vi "TestQtyCheck.vi"() -> ()   [LabVIEW 2012]
uses:
  <vilib>/addons/database/Auxilliary.llb/DB Tools Cursor Type.ctl
  <vilib>/Utility/NIReport.llb/NI_report.lvclass
  <vilib>/addons/database/Connection.llb/DB Tools Open Connec (Path).vi
  <vilib>/addons/database/Connection.llb/Conn Execute.vi
  <vilib>/addons/database/Recordset.llb/Rec Fetch Recordset Data (R).vi
  <vilib>/addons/database/Recordset.llb/Rec Destroy - Connection.vi
  <vilib>/addons/database/Recordset.llb/Rec Fetch Integer Data (R).vi
  <vilib>/addons/database/Recordset.llb/Rec Fetch String Data (R).vi
  <vilib>/Utility/NIReport.llb/Append Text Table to Report (wrap).vi
  <vilib>/addons/database/_DB Variant To Data/Database Variant To Data.xnode
  <vilib>/addons/database/NI_Database_API.lvlib
  <vilib>/Utility/NIReport.llb/Excel/NI_Excel.lvclass
panel:
  out "concatenated string 2":string
  out "error out 3":errorcluster
  out "error out 2":errorcluster
  in  "template (empty)":path=path "O:/Monitor/Report/機台報表示數量確認LIST.xls"
  out "array":string[][](array[string])
  out "spreadsheet string":string
  out "String":string
  out "concatenated string":string
  out "data":string
  out "data 4":i32
  out "data 3":string
  out "data 2":i32
  out "error out":errorcluster
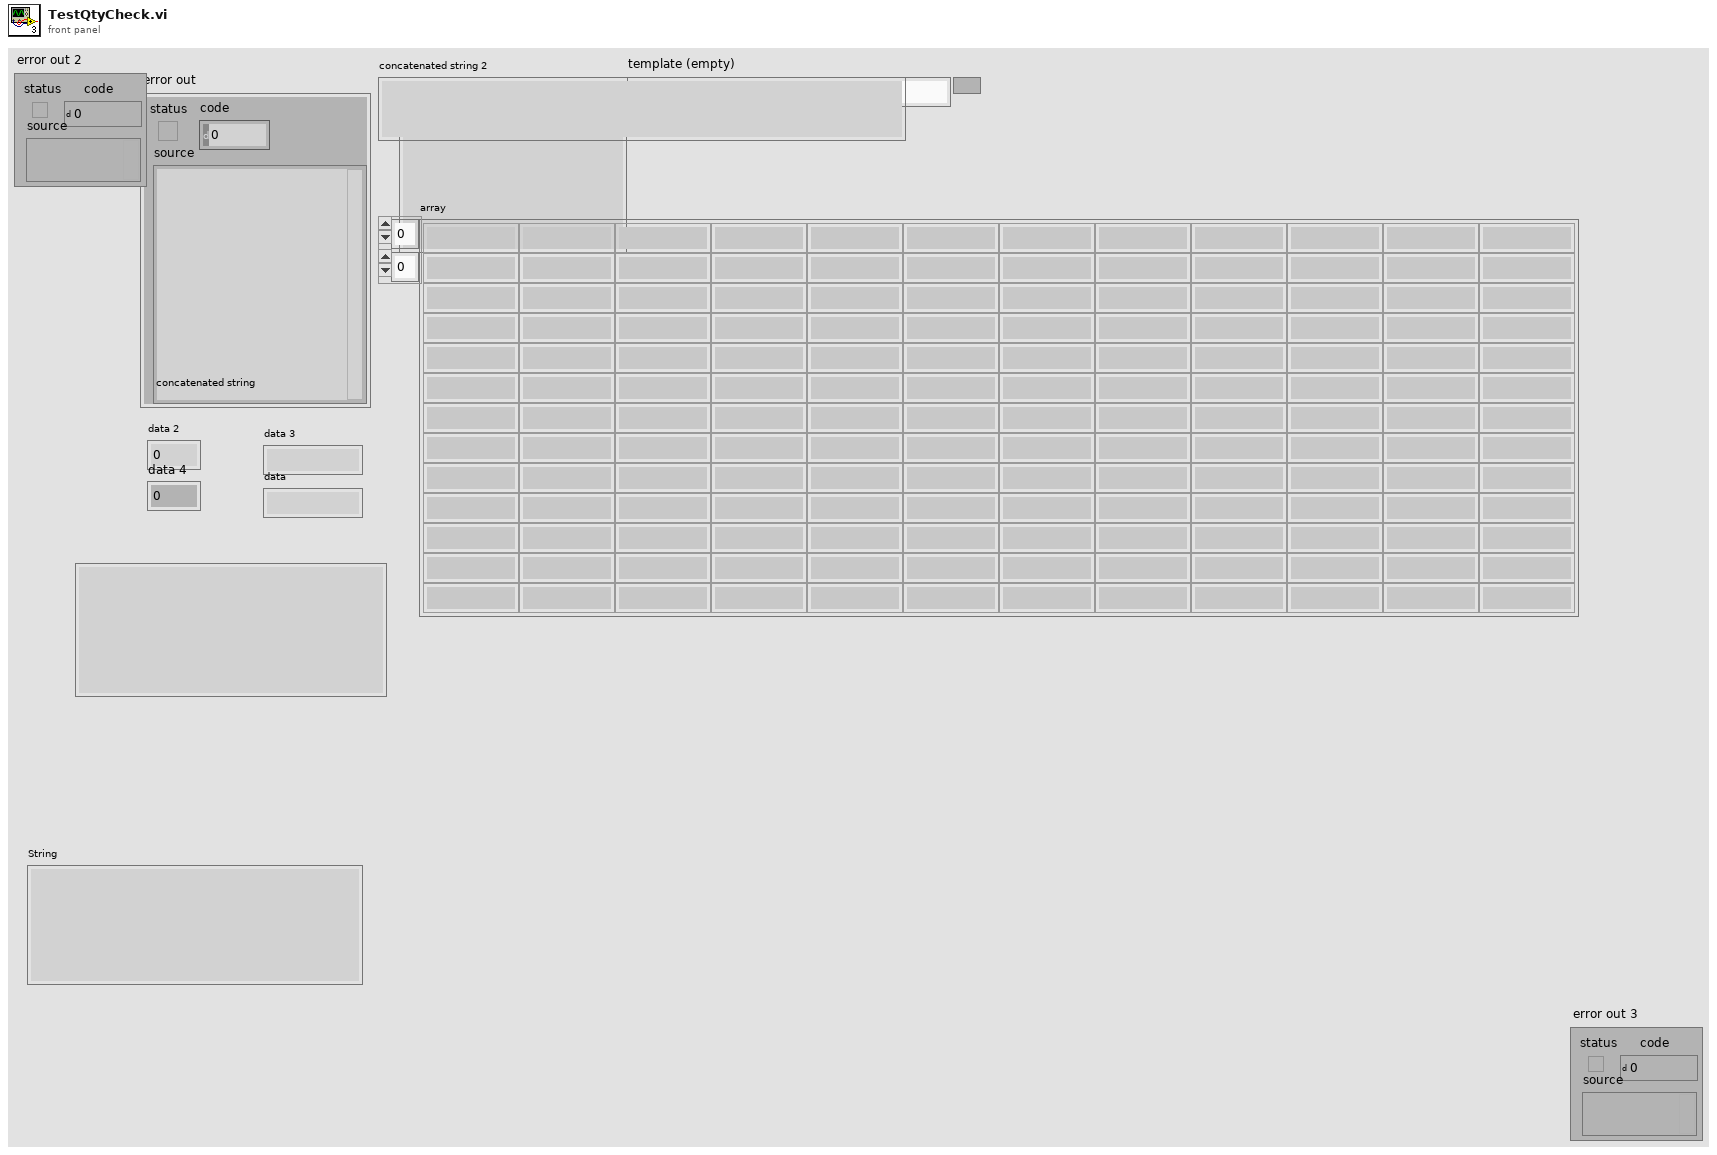
[diagram p1: front panel]
types:
  T1 = typedef "NI_Database_API.lvlib/DB Tools Cursor Type.ctl" = enum16{"forward-only", "keyset", "dynamic", "static"}
  T2 = typedef "NI_Database_API.lvlib/Conn ObjectReference.ctl" = refnum<k1>
  T3 = typedef "NI_Database_API.lvlib/Rec ObjectReference.ctl" = refnum<k1>
  T4 = enum16{"Standard Report", "HTML", "Word", "Excel"}
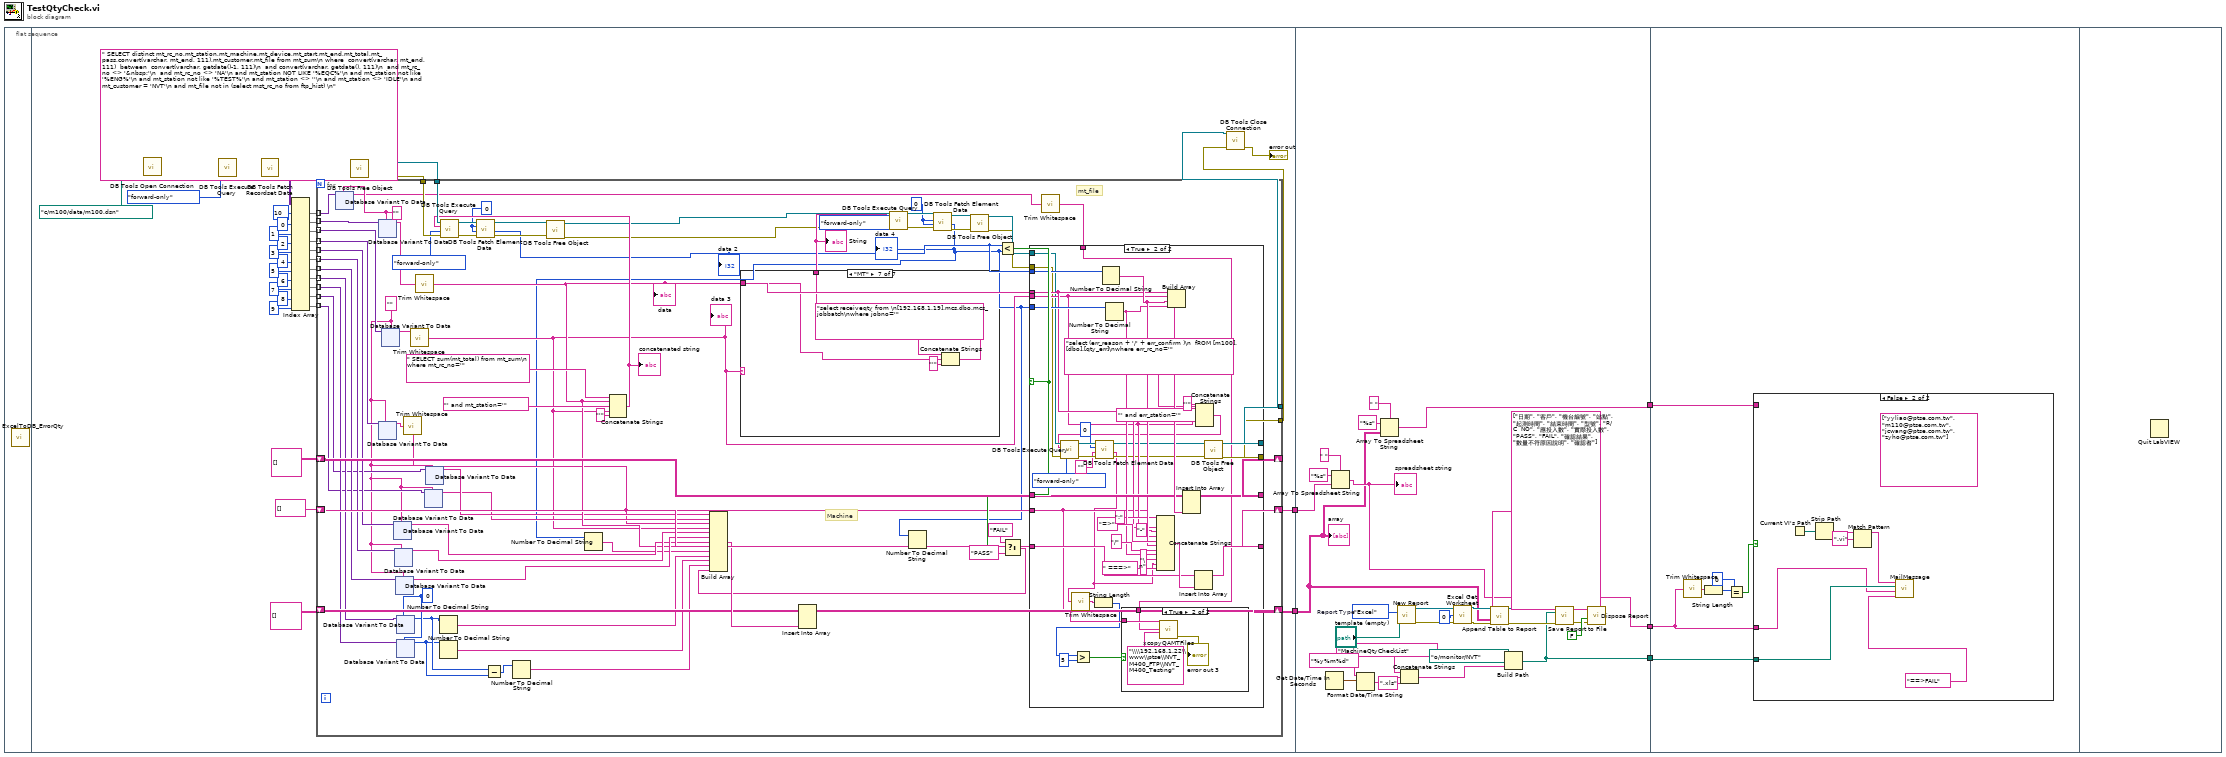
[diagram p0: block diagram]
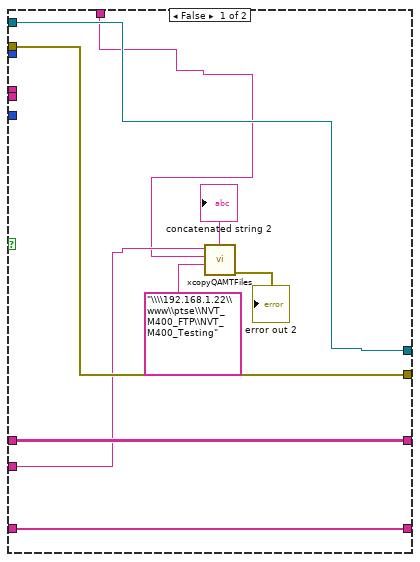
[diagram p2: hidden frame]
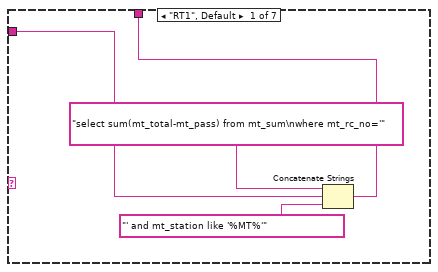
[diagram p4: hidden frame]
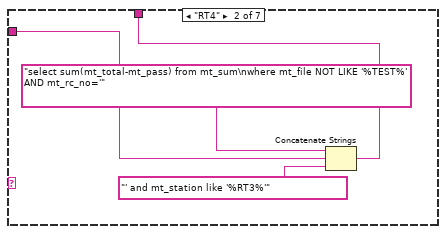
[diagram p5: hidden frame]
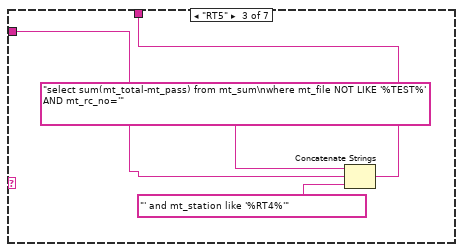
[diagram p6: hidden frame]
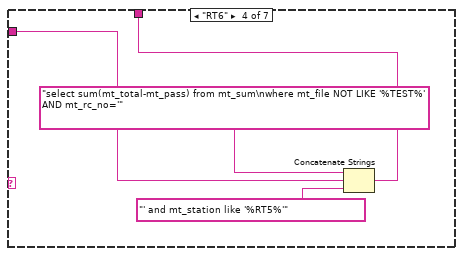
[diagram p7: hidden frame]
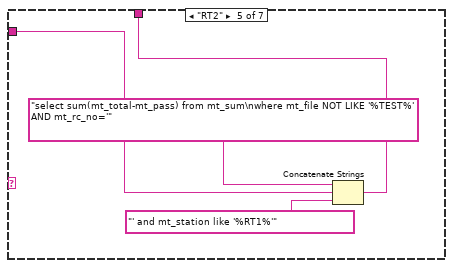
[diagram p8: hidden frame]
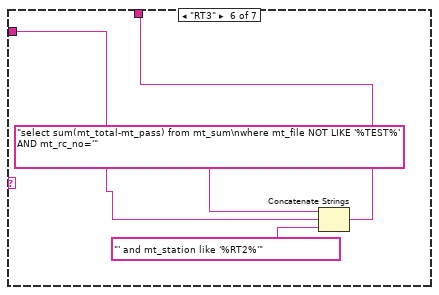
[diagram p9: hidden frame]
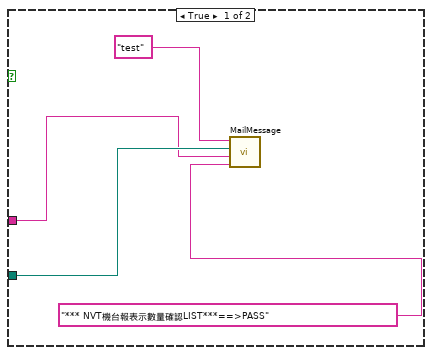
[diagram p10: hidden frame]
diagram:
  n1 = flat-sequence {
    tunnel: [w28] -> w5
    tunnel: [w24] -> w4
    tunnel: w5 -> [w579]
    tunnel: w4 -> [w555]
    tunnel: [w558] -> w3
    tunnel: [w557] -> w2
    tunnel: [w553] -> w1
    tunnel: w3 -> [w588]
    tunnel: w2 -> [w587]
    tunnel: w1 -> [w582]
    frame #0 {
      n2 = call "ExcelToDB_ErrorQty.vi"() -> ()  [unwired: 12 in]
    }
    frame #1 {
      n3 = call-poly <vilib>:"DB Tools Open Connection.vi"("connection information"=path "c:/m100/data/m100.dsn") -> ("error out"=w45:errorcluster, "connection reference"=w46:T2)  [unwired: 7 in]
      n4 = call-poly <vilib>:"DB Tools Execute Query.vi"("error in (no error)"=w45, "cursor type"=DB_Tools_Cursor_Type."forward-only", "SQL query"=" SELECT distinct mt_rc_no,mt_station,mt_machine,mt_device,mt_start,mt_end,mt_total,mt_pass,convert(varchar, mt_end, 111),mt_customer,mt_file from mt_sum\n where  convert(varchar, mt_end, 111)  between  convert(varchar, getdate()-1, 111)\n  and convert(varchar, getdate(), 111)\n  and mt_rc_no <> '&nbsp;'\n  and mt_rc_no <> 'NA'\n and mt_station NOT LIKE '%EQC%'\n and mt_station not like '%ENG%'\n and mt_station not like '%TEST%'\n and mt_station <> ''\n and mt_station <> 'IDLE'\n and mt_customer = 'NVT'\n and mt_file not in (select mst_rc_no from ftp_hist) \n", "connection reference"=w46) -> ("error out"=w43:errorcluster, "recordset reference"=w44:T3)  [unwired: 4 in]
      n5 = call-poly <vilib>:"DB Tools Fetch Recordset Data.vi"("error in (no error)"=w43, "recordset reference"=w44) -> ("error out"=w41:errorcluster, "recordset data"=w37:variant[][], "recordset reference out"=w42:T3)  [unwired: 3 in]
      n6 = Index Array(array=w37, index (col) #1=10 ("disabled index (col)"), index (col) #2=0 ("disabled index (col)"), index (col) #3=1 ("index (col)"), index (col) #4=2 ("index (col)"), index (col) #5=3 ("index (col)"), index (col) #6=4 ("index (col)"), index (col) #7=5 ("index (col)"), index (col) #8=6 ("index (col)"), index (col) #9=7 ("index (col)"), index (col) #10=8 ("index (col)"), index (col) #11=9 ("index (col)")) -> (element #1=w6:variant[], element #2=w36:variant[], element #3=w33:variant[], element #4=w26:variant[], element #5=w20:variant[], element #6=w19:variant[], element #7=w18:variant[], element #8=w15:variant[], element #9=w14:variant[], element #10=w11:variant[], element #11=w10:variant[])  [unwired: 11 in]
      n7 = call-poly <vilib>:"DB Tools Free Object.vi"("error in (no error)"=w41, "recordset reference"=w42) -> ("error out"=w31:errorcluster, "connection reference"=w32:T2)  [unwired: 8 in]
      n8 = for {
        tunnel: w36 -> [w111] mode=indexing
        tunnel: w33 -> [w119] mode=indexing
        tunnel: w32 -> [w110]
        tunnel: w31 -> [w109]
        shift-right: [w94] -> _
        shift-left: string[][] [] ("array") -> [w93]
        shift-right: [w54] -> w28
        shift-left: string[] [] ("array") -> [w92]
        tunnel: w26 -> [w91] mode=indexing
        shift-right: [w85] -> w24
        shift-left: string[][] [] ("array") -> [w83]
        tunnel: w20 -> [w82] mode=indexing
        tunnel: w19 -> [w81] mode=indexing
        tunnel: w18 -> [w80] mode=indexing
        tunnel: w15 -> [w79] mode=indexing
        tunnel: w14 -> [w78] mode=indexing
        tunnel: w11 -> [w73] mode=indexing
        tunnel: w10 -> [w72] mode=indexing
        tunnel: [w60] -> w9
        tunnel: [w59] -> w8
        tunnel: w6 -> [w58] mode=indexing
        w77 = 0
        w112 = 0
        w101 = 0
        w71 = ""
        w57 = ""
        # "Machine"
        # "mt_file"
        n9 = xnode "Database Variant To Data"("database variant"=w58, "type"=w57) -> ("data"=w56:string)  [unwired: 1 in, 1 out]
        n10 = xnode "Database Variant To Data"("database variant"=w91, "type"=w71) -> ("data"=w90:string)  [unwired: 1 in, 1 out]
        n11 = xnode "Database Variant To Data"("database variant"=w111, "type"=w57) -> ("data"=w95:string)  [unwired: 1 in, 1 out]
        n12 = xnode "Database Variant To Data"("database variant"=w119, "type"=w71) -> ("data"=w96:string)  [unwired: 1 in, 1 out]
        n13 = xnode "Database Variant To Data"("database variant"=w82, "type"=w71) -> ("data"=w68:string)  [unwired: 1 in, 1 out]
        n14 = xnode "Database Variant To Data"("database variant"=w81, "type"=w71) -> ("data"=w70:string)  [unwired: 1 in, 1 out]
        n15 = xnode "Database Variant To Data"("database variant"=w80, "type"=w71) -> ("data"=w69:string)  [unwired: 1 in, 1 out]
        n16 = xnode "Database Variant To Data"("database variant"=w79, "type"=w77) -> ("data"=w76:i32)  [unwired: 1 in, 1 out]
        n17 = xnode "Database Variant To Data"("database variant"=w78, "type"=w77) -> ("data"=w75:i32)  [unwired: 1 in, 1 out]
        n18 = call <vilib>:"Trim Whitespace.vi"("string"=w90) -> ("trimmed string"=w64:string)  [unwired: 1 in]
        n19 = call <vilib>:"Trim Whitespace.vi"("string"=w96) -> ("trimmed string"=w63:string)  [unwired: 1 in]
        "data 3" <- w63
        n20 = call <vilib>:"Trim Whitespace.vi"("string"=w95) -> ("trimmed string"=w67:string)  [unwired: 1 in]
        "data" <- w67
        n21 = xnode "Database Variant To Data"("database variant"=w72, "type"=w71) -> ("data"=w65:string)  [unwired: 1 in, 1 out]
        n22 = xnode "Database Variant To Data"("database variant"=w73, "type"=w71) -> ("data"=w66:string)  [unwired: 1 in, 1 out]
        n23 = Number To Decimal String(number=w76) -> (decimal integer string=w50:string)  [unwired: 1 in]
        n24 = Number To Decimal String(number=w75) -> (decimal integer string=w51:string)  [unwired: 1 in]
        n25 = Subtract(x=w76, y=w75) -> (x-y=w74:i32)
        n26 = Number To Decimal String(number=w74) -> (decimal integer string=w52:string)  [unwired: 1 in]
        n27 = Concatenate Strings(" SELECT sum(mt_total) from mt_sum\n where mt_rc_no='", w67, "' and mt_station='" ("string"), w63, "'" ("string")) -> (w102:string)
        "concatenated string" <- w102
        n28 = call-poly <vilib>:"DB Tools Execute Query.vi"("error in (no error)"=w109, "cursor type"=DB_Tools_Cursor_Type."forward-only", "SQL query"=w102, "connection reference"=w110) -> ("error out"=w107:errorcluster, "recordset reference"=w108:T3)  [unwired: 4 in]
        n29 = call-poly <vilib>:"DB Tools Fetch Element Data.vi"("error in (no error)"=w107, "type"=w101, "column index"=w101, "recordset reference"=w108) -> ("error out"=w99:errorcluster, "data"=w89:i32, "recordset reference out"=w100:T3)  [unwired: 3 in]
        "data 2" <- w89
        n30 = call-poly <vilib>:"DB Tools Free Object.vi"("error in (no error)"=w99, "recordset reference"=w100) -> ("error out"=w98:errorcluster, "connection reference"=w97:T2)  [unwired: 8 in]
        n31 = case shown="\"MT\"" w63 {
          tunnel: w67 -> [w462 w465 w469 w473 w478 w481 w487]
          tunnel: [w461 w466 w470 w474 w477 w482 w486] -> w114
          frame "RT1", Default {
            n32 = Concatenate Strings("select sum(mt_total-mt_pass) from mt_sum\nwhere mt_rc_no='" ("string"), w462, "' and mt_station like '%MT%'" ("string")) -> (w461:string)
          }
          frame "RT4" {
            n33 = Concatenate Strings("select sum(mt_total-mt_pass) from mt_sum\nwhere mt_file NOT LIKE '%TEST%' AND mt_rc_no='" ("string"), w465, "' and mt_station like '%RT3%'" ("string")) -> (w466:string)
          }
          frame "RT5" {
            n34 = Concatenate Strings("select sum(mt_total-mt_pass) from mt_sum\nwhere mt_file NOT LIKE '%TEST%' AND mt_rc_no='" ("string"), w469, "' and mt_station like '%RT4%'" ("string")) -> (w470:string)
          }
          frame "RT6" {
            n35 = Concatenate Strings("select sum(mt_total-mt_pass) from mt_sum\nwhere mt_file NOT LIKE '%TEST%' AND mt_rc_no='" ("string"), w473, "' and mt_station like '%RT5%'" ("string")) -> (w474:string)
          }
          frame "RT2" {
            n36 = Concatenate Strings("select sum(mt_total-mt_pass) from mt_sum\nwhere mt_file NOT LIKE '%TEST%' AND mt_rc_no='" ("string"), w478, "' and mt_station like '%RT1%'" ("string")) -> (w477:string)
          }
          frame "RT3" {
            n37 = Concatenate Strings("select sum(mt_total-mt_pass) from mt_sum\nwhere mt_file NOT LIKE '%TEST%' AND mt_rc_no='" ("string"), w481, "' and mt_station like '%RT2%'" ("string")) -> (w482:string)
          }
          frame "MT" {
            n38 = Concatenate Strings("select receiveqty from \n[192.168.1.19].mcs.dbo.mcs_jobbatch\nwhere jobno='" ("string"), w487, "'" ("string")) -> (w486:string)
          }
        }
        "String" <- w114
        n39 = call-poly <vilib>:"DB Tools Execute Query.vi"("error in (no error)"=w98, "cursor type"=DB_Tools_Cursor_Type."forward-only", "SQL query"=w114, "connection reference"=w97) -> ("error out"=w113:errorcluster, "recordset reference"=w117:T3)  [unwired: 4 in]
        n40 = call-poly <vilib>:"DB Tools Fetch Element Data.vi"("error in (no error)"=w113, "type"=w112, "column index"=w112, "recordset reference"=w117) -> ("error out"=w115:errorcluster, "data"=w49:i32, "recordset reference out"=w116:T3)  [unwired: 3 in]
        "data 4" <- w49
        n41 = Number To Decimal String(number=w49) -> (decimal integer string=w48:string)  [unwired: 1 in]
        n42 = Number To Decimal String(number=w49) -> ()  [unwired: 1 in, 1 out]
        n43 = call-poly <vilib>:"DB Tools Free Object.vi"("error in (no error)"=w115, "recordset reference"=w116) -> ("error out"=w61:errorcluster, "connection reference"=w62:T2)  [unwired: 8 in]
        n44 = Less?(x=w89, y=w49) -> (x < y?=w88:bool)
        n45 = Select(t="FAIL", s=w88, f="PASS") -> (s? t:f=w53:string)
        n46 = Build Array(w66, w65, w64, w63, w70, w69, w68, w67, w48, w50, w51, w52, w53) -> (w84:string[])
        n47 = Insert Into Array(array=w83, new element=w84) -> (w85:string[][])  [unwired: 2 in]
        n48 = call <vilib>:"Trim Whitespace.vi"("string"=w56) -> ("trimmed string"=w55:string)  [unwired: 1 in]
        n49 = case shown="True" w88 {
          tunnel: w67 -> [_ w441]
          tunnel: w63 -> [_ w439]
          tunnel: w89 -> [_ w456]
          tunnel: w49 -> [_ w455]
          tunnel: [w416 w453] -> w94
          tunnel: w93 -> [w416 w452]
          tunnel: [w415 w446] -> w54
          tunnel: w92 -> [w415 w445]
          tunnel: w64 -> [w412 w423]
          tunnel: w62 -> [w414 w433]
          tunnel: w61 -> [w413 w432]
          tunnel: [w414 w425] -> w60
          tunnel: [w413 w424] -> w59
          tunnel: w55 -> [w409 w422]
          frame False {
            n50 = call "xcopyQAMTFiles.vi"("Destination"="\\\\192.168.1.22\\www\\ptse\\NVT_M400_FTP\\NVT_M400_Testing", "SourceFile"=w409, "Machine"=w412) -> ("error out"=→"error out 2":errorcluster, "concatenated string"=→"concatenated string 2":string)  [unwired: 6 in]
          }
          frame True {
            n51 = Number To Decimal String(number=w456) -> (decimal integer string=w450:string)  [unwired: 1 in]
            n52 = Number To Decimal String(number=w455) -> (decimal integer string=w448:string)  [unwired: 1 in]
            n53 = Build Array(w441, w439, w450, w448) -> (w454:string[])
            n54 = Insert Into Array(array=w452, new element=w454) -> (w453:string[][])  [unwired: 2 in]
            n55 = Concatenate Strings("select (err_reason + '/' + err_confirm )\n  fROM [m100].[dbo].[qty_err]\nwhere err_rc_no='" ("string"), w441, "' and err_station='" ("string"), w439, "'" ("string")) -> (w430:string)
            n56 = call-poly <vilib>:"DB Tools Execute Query.vi"("error in (no error)"=w432, "cursor type"=DB_Tools_Cursor_Type."forward-only", "SQL query"=w430, "connection reference"=w433) -> ("error out"=w437:errorcluster, "recordset reference"=w436:T3)  [unwired: 4 in]
            n57 = call-poly <vilib>:"DB Tools Fetch Element Data.vi"("error in (no error)"=w437, "type"="", "column index"=0, "recordset reference"=w436) -> ("error out"=w434:errorcluster, "data"=w420:string, "recordset reference out"=w435:T3)  [unwired: 3 in]
            n58 = call <vilib>:"Trim Whitespace.vi"("string"=w420) -> ("trimmed string"=w421:string)  [unwired: 1 in]
            n59 = String Length(string=w421) -> (length=w419:i32)
            n60 = Greater?(x=w419, y=5) -> (0:w417:bool)
            n61 = case shown="True" w417 {
              tunnel: w423 -> [_ w458]
              tunnel: w422 -> [_ w457]
              frame False {
              }
              frame True {
                n62 = call "xcopyQAMTFiles.vi"("Destination"="\\\\192.168.1.22\\www\\ptse\\NVT_M400_FTP\\NVT_M400_Testing", "SourceFile"=w457, "Machine"=w458) -> ("error out"=→"error out 3":errorcluster)  [unwired: 6 in, 1 out]
              }
            }
            n63 = Concatenate Strings(w423, ":" ("string"), w441, "-" ("string"), w439, "=>" ("string"), w450, "/" ("string"), w448, " ===>" ("string"), w420, "\n" ("string")) -> (w447:string)
            n64 = Insert Into Array(array=w445, new element=w447) -> (w446:string[])  [unwired: 1 in]
            n65 = call-poly <vilib>:"DB Tools Free Object.vi"("error in (no error)"=w434, "recordset reference"=w435) -> ("error out"=w424:errorcluster, "connection reference"=w425:T2)  [unwired: 8 in]
          }
        }
      }
      n66 = call <vilib>:"DB Tools Close Connection.vi"("error in (no error)"=w8, "connection reference"=w9) -> ("error out"=→"error out":errorcluster)  [unwired: 5 in]
    }
    frame #2 {
      w578 = T4."Excel"  # Report Type
      n67 = Get Date/Time In Seconds() -> (seconds since 1Jan1904=w563:timestamp)
      n68 = Array To Spreadsheet String(delimiter (Tab)=" ", array=w579, 3:"%s" ("format string")) -> (spreadsheet string=w557:string)
      "spreadsheet string" <- w557
      n69 = Format Date/Time String(time format string (%c)="%y%m%d", seconds (now)=w563) -> (date/time string=w561:string)  [unwired: 1 in]
      n70 = Array To Spreadsheet String(delimiter (Tab)=" ", array=w555, 3:"%s" ("format string")) -> (spreadsheet string=w553:string)
      n71 = call <vilib>:"New Report.vi"("report type"=w578, "template (empty)"="template (empty)") -> ("report out"=w577:refnum<class "NI_report.lvclass">, "error out"=w576:errorcluster)  [unwired: 12 in]
      n72 = Concatenate Strings("MachineQtyCheckList" ("string"), w561, ".xls" ("string")) -> (w564:string)
      n73 = call <vilib>:"Excel Get Worksheet.vi"("report in"=w577, "worksheet index (0)"=0, "error in (no error)"=w576) -> ("report out"=w573:refnum<class "NI_report.lvclass">, "error out"=w572:errorcluster)  [unwired: 11 in]
      n74 = call-poly <vilib>:"Append Table to Report.vi"("report in"=w573, "column headers"=string[] ["日期", "客戶", "機台編號", "站點", "起測時間", "結束時間", "型號", "R/C  NO", "應投入數", "實際投入數", "PASS", "FAIL", "確認結果", "數量不符原因說明", "確認者"], "text data"=w555, "error in (no error)"=w572) -> ("report out"=w568:refnum<class "NI_report.lvclass">, "error out"=w567:errorcluster)  [unwired: 8 in, 2 out]
      n75 = Build Path(base path=path "o:/monitor/NVT", name or relative path=w564) -> (appended path=w558:path)
      n76 = call-dynamic "Save Report to File.vi"("report in"=w568, "report file path"=w558, "error in (no error)"=w567) -> ("report out"=w570:refnum<class "NI_report.lvclass">, "error out"=w569:errorcluster)  [unwired: 11 in]
      n77 = call-dynamic "Dispose Report.vi"("report in"=w570, "save changes? (F)"=FALSE, "error in (no error)"=w569) -> ()  [unwired: 12 in, 1 out]
      "array" <- w555
    }
    frame #3 {
      n78 = call <vilib>:"Trim Whitespace.vi"("string"=w587) -> ("trimmed string"=w586:string)  [unwired: 1 in]
      n79 = String Length(string=w586) -> (length=w585:i32)
      n80 = Equal?(x=w585, y=0) -> (x = y?=w583:bool)
      n81 = case shown="False" w583 {
        tunnel: w588 -> [w590 w595]
        tunnel: w587 -> [w589 w593]
        tunnel: w582 -> [_ _]
        frame True {
          n82 = call "MailMessage.vi"("AddSubject"="*** NVT機台報表示數量確認LIST***==>PASS" ("subject ([No Subject])"), "message"=w589, "file path"=w590, "program"="test") -> ()  [unwired: 8 in]
        }
        frame False {
          (unwired) string[] ["yyliao@ptse.com.tw", "m110@ptse.com.tw", "jcwang@ptse.com.tw", "zyho@ptse.com.tw"] ("recipients")
          n83 = Current VI's Path() -> (path=w599:path)
          n84 = Strip Path(path=w599) -> (name=w598:string)  [unwired: 1 out]
          n85 = Match Pattern(string=w598, regular expression=".vi") -> (before substring=w596:string)  [unwired: 1 in, 3 out]
          n86 = call "MailMessage.vi"("AddSubject"="==>FAIL" ("subject ([No Subject])"), "message"=w593, "file path"=w595, "program"=w596) -> ()  [unwired: 8 in]
        }
      }
    }
    frame #4 {
      n87 = Quit LabVIEW() -> ()  [unwired: 1 in]
    }
  }
